vi "add_EndEffectorCommand.vi"(3 "Position":sgl min=0 max=100, 4 "Commands":T1(ring), 5 "msg in":string) -> (2 "msg out":string)   [LabVIEW 2012]
doc: "Flattens end effector commands into a string"
uses:
  <userlib>/ROS for LabVIEW Software/ROS/MessageBuilding/std_msgs/subs/u32Scalar.vi
  <userlib>/ROS for LabVIEW Software/ROS/MessageBuilding/std_msgs/subs/stringScalar.vi
panel:
  # "Known Accepted Commands at this point are\n     - Calibrate\n     - Clear Calibration\n     - Go (uses Position)"
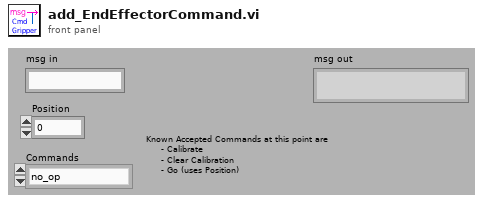
[diagram p1: front panel]
types:
  T1 = enum16{"no_op", "set", "configure", "reboot", "reset", "calibrate", "clear_calibration", "prepare_to_grip", "grip", "release", "go", "stop"}
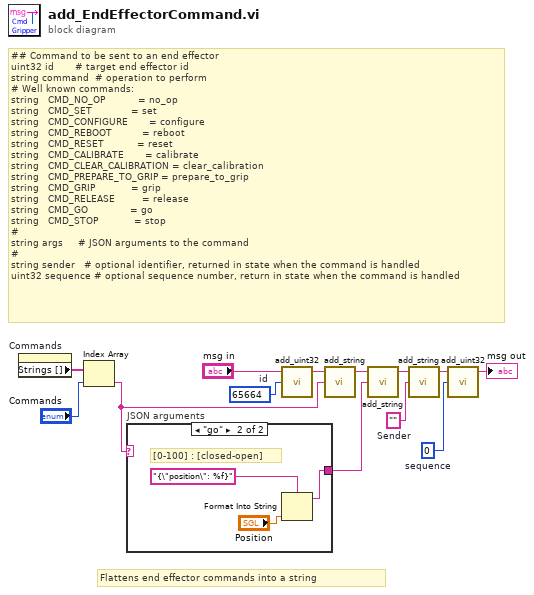
[diagram p0: block diagram]
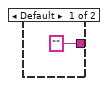
[diagram p2: hidden frame]
diagram:
  w3 = u32 0  # sequence
  w4 = ""  # Sender
  w12 = u32 65664  # id
  # "Flattens end effector commands into a string"
  # "## Command to be sent to an end effector\nuint32 id       # target end effector id\nstring command  # operation to perform\n# Well known commands:\nstring   CMD_NO_OP           = no_op\nstring   CMD_SET             = set\nstring   CMD_CONFIGURE       = configure\nstring   CMD_REBOOT          = reboot\nstring   CMD_RESET           = reset\nstring   CMD_CALIBRATE       = calibrate\nstring   CMD_CLEAR_CALIBRATION = clear_calibration\nstring   CMD_PREPARE_TO_GRIP = prepare_to_grip\nstring   CMD_GRIP            = grip\nstring   CMD_RELEASE         = release\nstring   CMD_GO              = go\nstring   CMD_STOP            = stop\n#\nstring args     # JSON arguments to the command\n#\nstring sender   # optional identifier, returned in state when the command is handled\nuint32 sequence # optional sequence number, return in state when the command is handled"
  n1 = property on="Commands" class="Enum (strict)"() -> ("Strings []"=w11:string[])  [unwired: 2 in, 2 out]
  n2 = Index Array(array=w11, index="Commands") -> (element=w1:string)
  n3 = case "JSON arguments" shown="\"go\"" w1 {
    tunnel: ["" ("String") w15] -> w9
    frame Default {
    }
    frame "go" {
      # "[0-100] : [closed-open]"
      n4 = Format Into String(format string="{\"position\": %f}", "Position") -> (resulting string=w15:string)  [unwired: 2 in, 1 out]
    }
  }
  n5 = call-poly <userlib>:"add_uint32.vi"("Numeric"=w12, "msg in"="msg in") -> ("msg out"=w13:string)  [unwired: 3 in]
  n6 = call-poly <userlib>:"add_string.vi"("String"=w1, "msg in"=w13) -> ("msg out"=w10:string)  [unwired: 3 in]
  n7 = call-poly <userlib>:"add_string.vi"("String"=w9, "msg in"=w10) -> ("msg out"=w7:string)  [unwired: 3 in]
  n8 = call-poly <userlib>:"add_string.vi"("String"=w4, "msg in"=w7) -> ("msg out"=w6:string)  [unwired: 3 in]
  n9 = call-poly <userlib>:"add_uint32.vi"("Numeric"=w3, "msg in"=w6) -> ("msg out"=→"msg out":string)  [unwired: 3 in]
